vi "Generate slice pattern.vi"(9 "thin slice (um)":dbl=100.0 format="%#_13g", 10 "thick slice (um)":dbl=500.0 format="%#_13g", 11 "repitition":i32=14) -> (1 "Array":dbl[](array[numeric]))   [LabVIEW 2017]
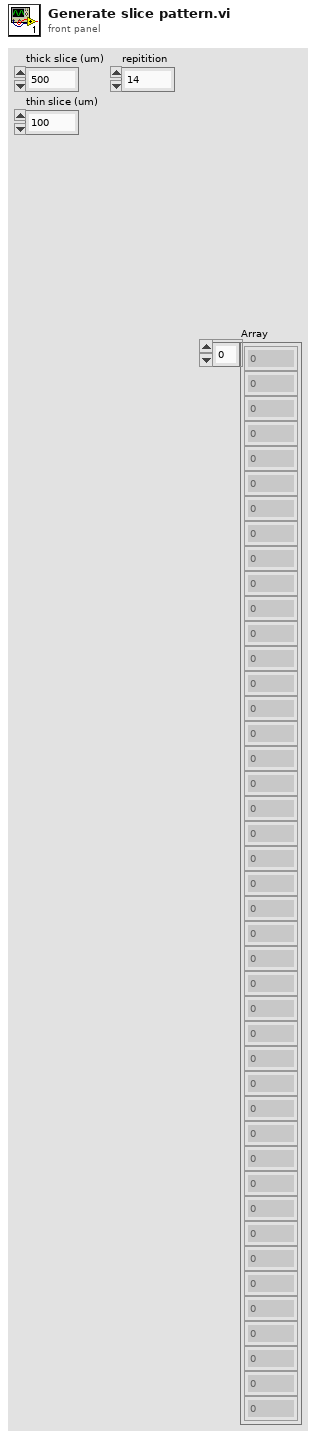
[diagram p1: front panel]
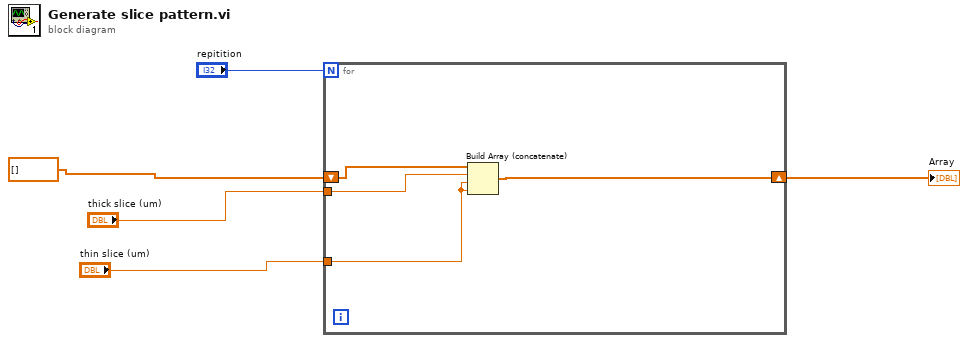
[diagram p0: block diagram]
diagram:
  n1 = for {
    N: "repitition" -> [_]
    shift-right: [w8] -> w1
    shift-left: dbl[] [] ("element") -> [w9]
    tunnel: "thick slice (um)" -> [w7]
    tunnel: "thin slice (um)" -> [w6]
    n2 = Build Array (concatenate)(w9, w7, w6, w6) -> (w8:dbl[])
  }
  "Array" <- w1
